vi "MAR!.vi"(0 "System no.":i32=1 min=1 max=4 step=1, 2 "Move mode":u16(ring)=2 items=["Move X", "Move Y", "Move Z", "Move U", "Move V", "Move W", "Move XY", "Move XZ", "Move XU", "Move XV", "Move XW", "Move YZ", "Move YU", "Move YV", "Move YW", "Move ZU", "Move ZV", "Move ZW", "Move UV", "Move UW", "Move VW", "Move XYZ", "Move UVW", "Move XYZUVW"], 3 "Translation":cluster{"X":dbl, "Y":dbl, "Z":dbl} {"Z" format="%.4f"; "Y" format="%.4f"; "X" format="%.4f"}, 4 "Rotation":cluster{"U":dbl, "V":dbl, "W":dbl} {"W" format="%.4f"; "V" format="%.4f"; "U" format="%.4f"}, 5 "error in":errorcluster) -> (14 "Motion started":bool, 15 "Motion stopped":bool, 19 "error out":errorcluster)   [LabVIEW 2020]
doc: "M-8X0-specific command. Moves stage. Waits for M-8X0 controller to reply 1 when all calculations are done and the movement starts, and another 1 when motion is complete.\n\nC-887, M-8X0: Only for GCS syntax version = GCS 1.0 (Check with CSV?.vi. If CSV?.vi is not supported, syntax version is GCS 1.0). For compatibility, calls MOV.vi for GCS 2.0 or higher (in this case Motion started returns TRUE immediately, Motion stopped is determined by #5 polling."
uses:
  Controller names.ctl
  Syntax.ctl
  Global2 (Array).vi
  Global1.vi
panel:
  # "M-850 specific command. Moves stage. Waits for M-850 controller\nto reply 1 when all calculations are done and the movement starts,\nand another 1 when motion is complete."
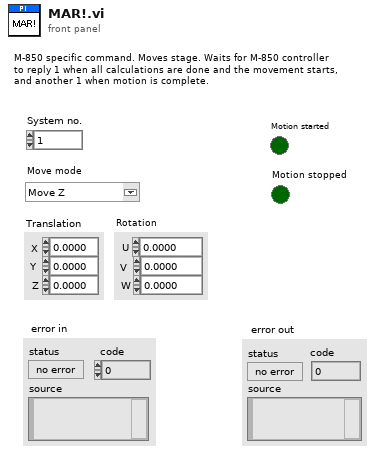
[diagram p1: front panel]
types:
  T1 = typedef "Syntax.ctl" = enum16{"GCS 1.0", "GCS 2.0", "GCS 3.0"}
  T2 = typedef "Controller names.ctl" = enum16{"None", "Analog", "C-702", "C-413", "C-414", "C-843", "C-843.PM", "C-844", "C-848", "C-865", "C-866", "C-867", "C-877", "C-880", "C-884", "C-885", "C-886", "C-887", "C-891", "E-135", "E-516", "E-517", "E-518", "E-709", "E-710", "E-712", "E-725", "E-727", "E-753", "E-754", "E-755", "E-761", "E-816", "E-861", "E-870", "E-871", "E-872", "E-873", "E-874", "F-206", "HydraPollux", "M-840", "M-850", "M-8X0", "Mercury", "Mercury_GCS", "PI_GCS2"}
  T3 = cluster{"Conn. axes":string[], "Controller name":T2}[]
  T4 = cluster{"Conn. axes":string[], "Controller name":T2}
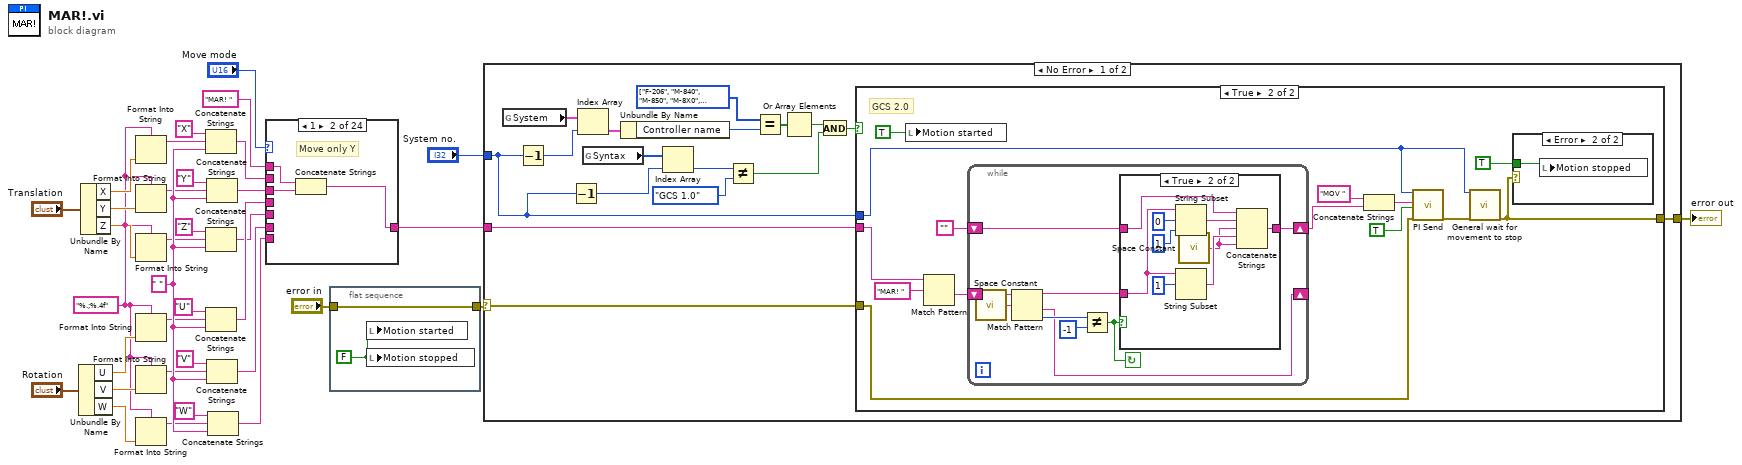
[diagram p0: block diagram]
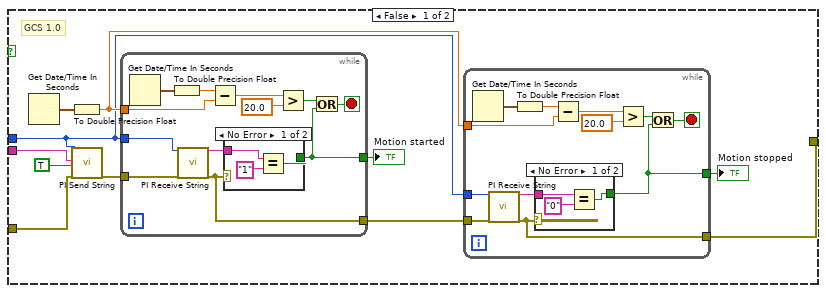
[diagram p2: hidden frame]
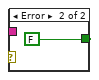
[diagram p3: hidden frame]
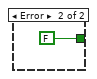
[diagram p4: hidden frame]
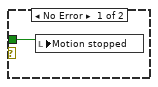
[diagram p6: hidden frame]
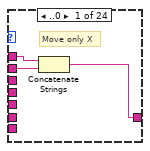
[diagram p8: hidden frame]
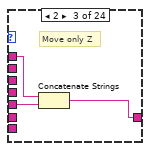
[diagram p9: hidden frame]
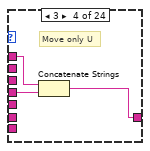
[diagram p10: hidden frame]
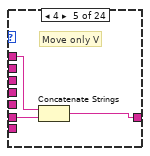
[diagram p11: hidden frame]
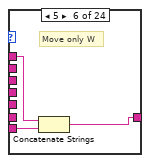
[diagram p12: hidden frame]
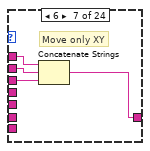
[diagram p13: hidden frame]
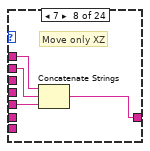
[diagram p14: hidden frame]
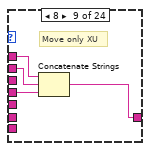
[diagram p15: hidden frame]
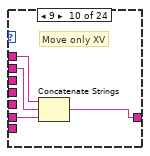
[diagram p16: hidden frame]
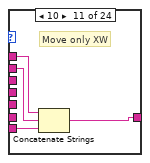
[diagram p17: hidden frame]
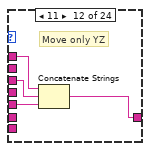
[diagram p18: hidden frame]
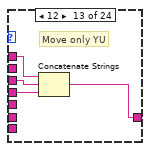
[diagram p19: hidden frame]
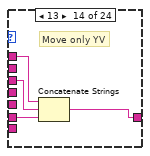
[diagram p20: hidden frame]
diagram:
  w6 = "%.;%.4f" ("Format String")
  w28 = " "
  n1 = Unbundle By Name("Rotation") -> ("U"=w9:dbl, "V"=w8:dbl, "W"=w7:dbl)
  n2 = Unbundle By Name("Translation") -> ("X"=w18:dbl, "Y"=w11:dbl, "Z"=w10:dbl)
  n3 = Format Into String(format string=w6, w18) -> (resulting string=w17:string)  [unwired: 2 in, 1 out]
  n4 = Format Into String(format string=w6, w11) -> (resulting string=w16:string)  [unwired: 2 in, 1 out]
  n5 = Format Into String(format string=w6, w10) -> (resulting string=w15:string)  [unwired: 2 in, 1 out]
  n6 = Format Into String(format string=w6, w9) -> (resulting string=w14:string)  [unwired: 2 in, 1 out]
  n7 = Format Into String(format string=w6, w8) -> (resulting string=w13:string)  [unwired: 2 in, 1 out]
  n8 = Format Into String(format string=w6, w7) -> (resulting string=w12:string)  [unwired: 2 in, 1 out]
  n9 = Concatenate Strings("X", w17, w28) -> (w31:string)
  n10 = Concatenate Strings("Z", w15, w28) -> (w26:string)
  n11 = Concatenate Strings("U", w14, w28) -> (w27:string)
  n12 = Concatenate Strings("Y", w16, w28) -> (w25:string)
  n13 = Concatenate Strings("V", w13, w28) -> (w29:string)
  n14 = Concatenate Strings("W", w12, w28) -> (w30:string)
  n15 = case shown="1" "Move mode" {
    tunnel: w31 -> [w37 _ _ _ _ _ w55 w59 w63 w67 w72 _ _ _ _ _ _ _ _ _ _ w116 _ w129]
    tunnel: "MAR! " -> [w38 w41 w44 w47 w50 w53 w57 w61 w65 w69 w73 w77 w81 w85 w89 w93 w97 w101 w105 w109 w113 w118 w123 w131]
    tunnel: [w36 w40 w43 w46 w49 w52 w56 w60 w64 w68 w70 w76 w80 w84 w88 w92 w96 w100 w104 w108 w112 w117 w122 w130] -> w5
    tunnel: w30 -> [_ _ _ _ _ w51 _ _ _ _ w71 _ _ _ w86 _ _ w98 _ w106 w111 _ w119 w124]
    tunnel: w29 -> [_ _ _ _ w48 _ _ _ _ w66 _ _ _ w82 _ _ w94 _ w102 _ w110 _ w120 w125]
    tunnel: w27 -> [_ _ _ w45 _ _ _ _ w62 _ _ _ w78 _ _ w90 _ _ w103 w107 _ _ w121 w126]
    tunnel: w26 -> [_ _ w42 _ _ _ _ w58 _ _ _ w74 _ _ _ w91 w95 w99 _ _ _ w114 _ w127]
    tunnel: w25 -> [_ w39 _ _ _ _ w54 _ _ _ _ w75 w79 w83 w87 _ _ _ _ _ _ w115 _ w128]
    frame ..0 {
      # "Move only X"
      n16 = Concatenate Strings(w38, w37) -> (w36:string)
    }
    frame 1 {
      # "Move only Y"
      n17 = Concatenate Strings(w41, w39) -> (w40:string)
    }
    frame 2 {
      # "Move only Z"
      n18 = Concatenate Strings(w44, w42) -> (w43:string)
    }
    frame 3 {
      # "Move only U"
      n19 = Concatenate Strings(w47, w45) -> (w46:string)
    }
    frame 4 {
      # "Move only V"
      n20 = Concatenate Strings(w50, w48) -> (w49:string)
    }
    frame 5 {
      # "Move only W"
      n21 = Concatenate Strings(w53, w51) -> (w52:string)
    }
    frame 6 {
      # "Move only XY"
      n22 = Concatenate Strings(w57, w55, w54) -> (w56:string)
    }
    frame 7 {
      # "Move only XZ"
      n23 = Concatenate Strings(w61, w59, w58) -> (w60:string)
    }
    frame 8 {
      # "Move only XU"
      n24 = Concatenate Strings(w65, w63, w62) -> (w64:string)
    }
    frame 9 {
      # "Move only XV"
      n25 = Concatenate Strings(w69, w67, w66) -> (w68:string)
    }
    frame 10 {
      # "Move only XW"
      n26 = Concatenate Strings(w73, w72, w71) -> (w70:string)
    }
    frame 11 {
      # "Move only YZ"
      n27 = Concatenate Strings(w77, w75, w74) -> (w76:string)
    }
    frame 12 {
      # "Move only YU"
      n28 = Concatenate Strings(w81, w79, w78) -> (w80:string)
    }
    frame 13 {
      # "Move only YV"
      n29 = Concatenate Strings(w85, w83, w82) -> (w84:string)
    }
    frame 14 {
      # "Move only YW"
      n30 = Concatenate Strings(w89, w87, w86) -> (w88:string)
    }
    frame 15 {
      # "Move only ZU"
      n31 = Concatenate Strings(w93, w91, w90) -> (w92:string)
    }
    frame 16 {
      # "Move only ZV"
      n32 = Concatenate Strings(w97, w95, w94) -> (w96:string)
    }
    frame 17 {
      # "Move only ZW"
      n33 = Concatenate Strings(w101, w99, w98) -> (w100:string)
    }
    frame 18 {
      # "Move only UV"
      n34 = Concatenate Strings(w105, w103, w102) -> (w104:string)
    }
    frame 19 {
      # "Move only UW"
      n35 = Concatenate Strings(w109, w107, w106) -> (w108:string)
    }
    frame 20 {
      # "Move only VW"
      n36 = Concatenate Strings(w113, w110, w111) -> (w112:string)
    }
    frame 21 {
      # "Move only XYZ"
      n37 = Concatenate Strings(w118, w116, w115, w114) -> (w117:string)
    }
    frame 22 {
      # "Move only UVW"
      n38 = Concatenate Strings(w123, w121, w120, w119) -> (w122:string)
    }
    frame 23.. {
      # "Move XYZ UVW"
      n39 = Concatenate Strings(w131, w129, w128, w127, w126, w125, w124) -> (w130:string)
    }
  }
  n40 = flat-sequence {
    tunnel: [w132] -> w1
    tunnel: "error in" -> [w132]
    frame #0 {
      w133 = FALSE ("Motion started")
      n41 = local write "Motion started"(w133) -> ()
      n42 = local write "Motion stopped"(w133) -> ()
    }
  }
  n43 = case shown="No Error" w1 {
    selector: w1 -> [w135 w229]
    tunnel: w5 -> [w150 _]
    tunnel: [w149 w229] -> w4
    tunnel: "System no." -> [w139 _]
    frame No Error {
      w147 = T2[] [enum."F-206", enum."M-840", enum."M-850", enum."M-8X0", enum."C-887"] items=["None", "Analog", "C-702", "C-413", "C-414", "C-843", "C-843.PM", "C-844", "C-848", "C-865", "C-866", "C-867", "C-877", "C-880", "C-884", "C-885", "C-886", "C-887", "C-891", "E-135", "E-516", "E-517", "E-518", "E-709", "E-710", "E-712", "E-725", "E-727", "E-753", "E-754", "E-755", "E-761", "E-816", "E-861", "E-870", "E-871", "E-872", "E-873", "E-874", "F-206", "HydraPollux", "M-840", "M-850", "M-8X0", "Mercury", "Mercury_GCS", "PI_GCS2"]
      n44 = global read "Global2 (Array).vi" "System"() -> (w144:T3)
      n45 = Decrement(x=w139) -> (x-1=w136:i32)
      n46 = Decrement(x=w139) -> (x-1=w142:i32)
      n47 = Index Array(array=w144, index=w136) -> (element=w145:T4)
      n48 = global read "Global1.vi" "Syntax"() -> (w143:T1[])
      n49 = Unbundle By Name(w145) -> ("Controller name"=w146:T2)
      n50 = Index Array(array=w143, index=w142) -> (element=w141:T1)
      n51 = Not Equal?(x=w141, y=Syntax."GCS 1.0") -> (x != y?=w140:bool)
      n52 = Equal?(x=w147, y=w146) -> (x = y?=w148:bool[])
      n53 = Or Array Elements(Boolean array=w148) -> (logical OR=w138:bool)
      n54 = And(x=w138, y=w140) -> (x .and. y?=w137:bool)
      n55 = case shown="True" w137 {
        tunnel: w135 -> [w161 w202]
        tunnel: w150 -> [w159 w201]
        tunnel: [w157 w194] -> w149
        tunnel: w139 -> [w155 w203]
        frame False {
          # "GCS 1.0"
          n56 = Get Date/Time In Seconds() -> (seconds since 1Jan1904=w153:timestamp)
          n57 = To Double Precision Float(number=w153) -> (double precision float=w156:dbl)
          n58 = call "PI Send String.vi"("System no."=w155, "String to send"=w159, "Attach termination char.?"=TRUE ("Attach Linefeed?"), "error in"=w161) -> ("error out"=w154:errorcluster)  [unwired: 15 out]
          n59 = while {
            tunnel: [w165] -> w151
            tunnel: [w162] -> w158
            tunnel: w156 -> [w169]
            tunnel: w154 -> [w171]
            tunnel: w155 -> [w172]
            stop <- w163 stop-if-true
            n60 = Get Date/Time In Seconds() -> (seconds since 1Jan1904=w164:timestamp)
            n61 = To Double Precision Float(number=w164) -> (double precision float=w170:dbl)
            n62 = call "PI Receive String.vi"("System no."=w172, "error in"=w171) -> ("String read"=w173:string, "error out"=w162:errorcluster)  [unwired: 1 in, 15 out]
            n63 = Subtract(x=w170, y=w169) -> (x-y=w168:dbl)
            n64 = case shown="No Error" w162 {
              tunnel: w173 -> [w176 _]
              tunnel: [w175 FALSE] -> w165
              frame No Error {
                n65 = Equal?(x=w176, y="1") -> (x = y?=w175:bool)
              }
              frame Error {
              }
            }
            n66 = Greater?(x=w168, y=20.0) -> (0:w166:bool)
            n67 = Or(x=w166, y=w165) -> (x .or. y?=w163:bool)
          }
          "Motion started" <- w151
          n68 = while {
            tunnel: [w181] -> w152
            tunnel: [w179] -> w157
            tunnel: w156 -> [w185]
            tunnel: w158 -> [w187]
            tunnel: w155 -> [w188]
            stop <- w178 stop-if-true
            n69 = Get Date/Time In Seconds() -> (seconds since 1Jan1904=w180:timestamp)
            n70 = call "PI Receive String.vi"("System no."=w188, "error in"=w187) -> ("String read"=w189:string, "error out"=w179:errorcluster)  [unwired: 1 in, 15 out]
            n71 = To Double Precision Float(number=w180) -> (double precision float=w186:dbl)
            n72 = case shown="No Error" w179 {
              tunnel: w189 -> [w192 _]
              tunnel: [w191 FALSE] -> w181
              frame No Error {
                n73 = Equal?(x=w192, y="0") -> (x = y?=w191:bool)
              }
              frame Error {
              }
            }
            n74 = Subtract(x=w186, y=w185) -> (x-y=w184:dbl)
            n75 = Greater?(x=w184, y=20.0) -> (0:w182:bool)
            n76 = Or(x=w182, y=w181) -> (x .or. y?=w178:bool)
          }
          "Motion stopped" <- w152
        }
        frame True {
          # "GCS 2.0"
          n77 = local write "Motion started"(TRUE) -> ()
          n78 = Match Pattern(string=w201, regular expression="MAR! ") -> (after substring=w198:string)  [unwired: 4 out]
          n79 = while {
            shift-right: [w208] -> _
            shift-left: w198 -> [w213]
            shift-right: [w212] -> w196
            shift-left: "" -> [w210]
            stop <- w214 continue-if-true
            n80 = call "Space Constant.vi"() -> ("String"=w216:string)
            n81 = Match Pattern(string=w213, regular expression=w216) -> (before substring=w209:string, after substring=w208:string, offset past match=w215:i32)  [unwired: 2 out]
            n82 = Not Equal?(x=w215, y=-1) -> (x != y?=w214:bool)
            n83 = case shown="True" w214 {
              tunnel: w209 -> [_ w223]
              tunnel: [w217 w225] -> w212
              tunnel: w210 -> [w217 w219]
              frame False {
              }
              frame True {
                n84 = String Subset(string=w223, offset (0)=0, length (rest)=1 ("length (rest)")) -> (substring=w222:string)
                n85 = String Subset(string=w223, offset (0)=1) -> (substring=w220:string)  [unwired: 1 out]
                n86 = call "Space Constant.vi"() -> ("String"=w218:string)
                n87 = Concatenate Strings(w219, w222, w218, w220, w218) -> (w225:string)
              }
            }
          }
          n88 = Concatenate Strings("MOV ", w196) -> (w195:string)
          n89 = call "PI Send.vi"("System no."=w203, "String to send"=w195, "Attach termination char.?"=TRUE ("Attach Linefeed?"), "error in"=w202) -> ("error out"=w204:errorcluster)  [unwired: 2 in, 13 out]
          n90 = call "General wait for movement to stop.vi"("System no."=w203, "error in"=w204) -> ("error out"=w194:errorcluster)  [unwired: 6 in, 11 out]
          n91 = case shown="Error" w194 {
            tunnel: TRUE ("Motion stopped") -> [w227 w228]
            frame No Error {
              n92 = local write "Motion stopped"(w227) -> ()
            }
            frame Error {
              n93 = local write "Motion stopped"(w228) -> ()
            }
          }
        }
      }
    }
    frame Error {
    }
  }
  "error out" <- w4
